vi "(SubVI) SaveTxtHeader.vi"(0 "Frames":u32, 1 "Folder Path":path, 2 "Width (pixell)":i32, 3 "Height (pixell)":i32, 4 "pixel_depth":i16, 5 "avg_fps (Hz)":dbl) -> (6 "saved path":path, 7 "Header":string[][](array[string]))   [LabVIEW 2014]
uses:
  <vilib>/Utility/file.llb/Write To Spreadsheet File (string).vi
panel:
  in  "Select a Folder":path
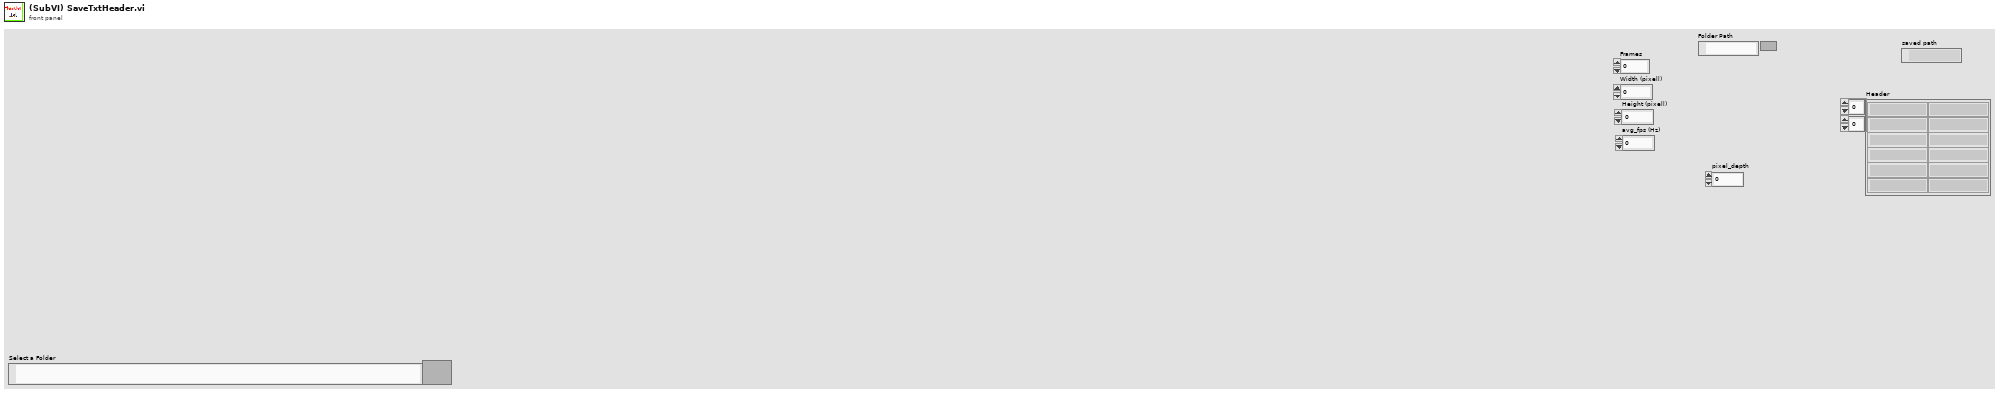
[diagram p1: front panel]
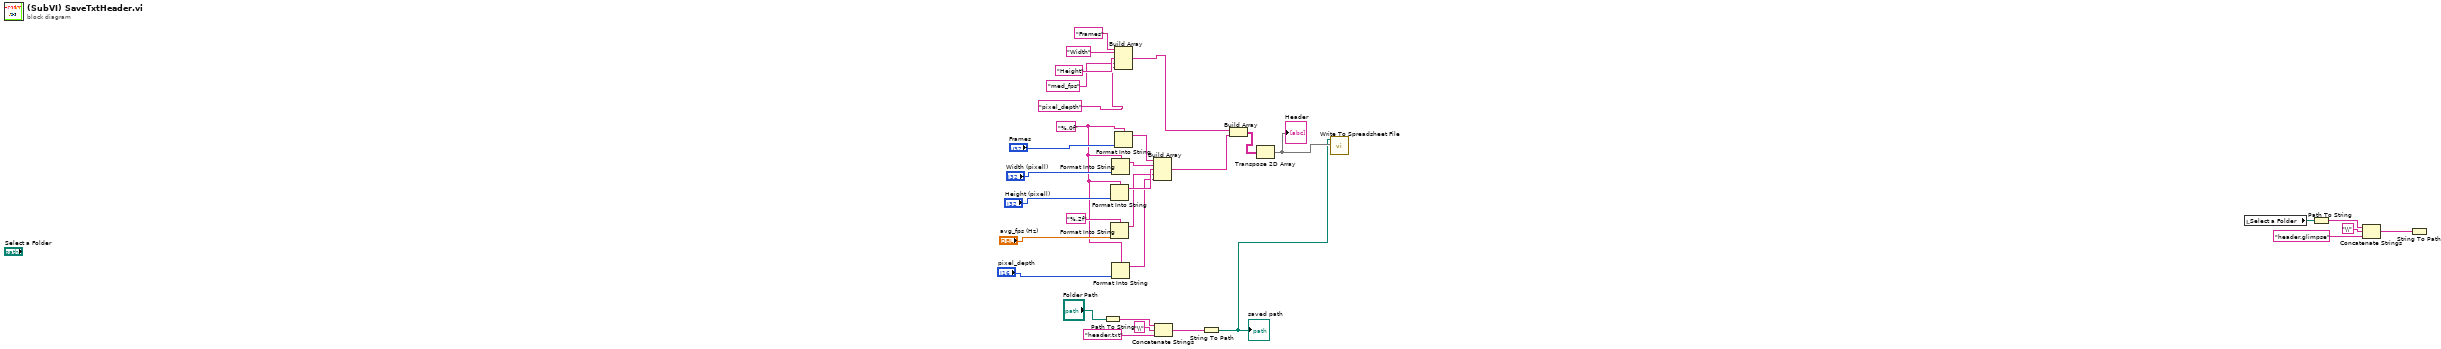
[diagram p0: block diagram]
diagram:
  w18 = "%.0f" ("initial string")
  n1 = Path To String(path="Folder Path") -> (string=w6:string)
  n2 = Format Into String(format string=w18, "Height (pixell)") -> (resulting string=w22:string)  [unwired: 2 in, 1 out]
  n3 = Format Into String(format string="%.2f" ("initial string"), "avg_fps (Hz)") -> (resulting string=w19:string)  [unwired: 2 in, 1 out]
  n4 = Format Into String(format string=w18, "Width (pixell)") -> (resulting string=w24:string)  [unwired: 2 in, 1 out]
  n5 = Format Into String(format string=w18, "pixel_depth") -> (resulting string=w16:string)  [unwired: 2 in, 1 out]
  n6 = Build Array("Frames" ("string"), "Width" ("string"), "Height" ("string"), "med_fps" ("string"), "pixel_depth" ("string")) -> (w15:string[])
  n7 = Format Into String(format string=w18, "Frames") -> (resulting string=w26:string)  [unwired: 2 in, 1 out]
  n8 = Build Array(w26, w24, w22, w19, w16) -> (w14:string[])
  n9 = Concatenate Strings(w6, "\\" ("string"), "header.txt" ("string")) -> (w5:string)
  n10 = String To Path(string=w5) -> (path=w1:path)
  "saved path" <- w1
  n11 = Build Array(w15, w14) -> (w13:string[][])
  n12 = Transpose 2D Array(2D array=w13) -> (transposed array=w2:string[][])
  "Header" <- w2
  n13 = call-poly <vilib>:"Write To Spreadsheet File.vi"("2D data"=w2, "file path (dialog if empty)"=w1) -> ()  [unwired: 6 in, 1 out]
  n14 = local read "Select a Folder"() -> (w12:path)
  n15 = Path To String(path=w12) -> (string=w10:string)
  n16 = Concatenate Strings(w10, "\\" ("string"), "header.glimpse" ("string")) -> (w9:string)
  n17 = String To Path(string=w9) -> ()  [unwired: 1 out]
